vi "Kinetics camera control 1.vi"() -> ()   [LabVIEW 2020]
uses:
  C:/Users/Public/Documents/Photometrics/PMQI-LabViewSamples/Examples/2018/Dependencies/PVCamNET.dll
  PVCamNET.dll
panel:
  in  "stop":bool
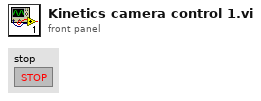
[diagram p1: front panel]
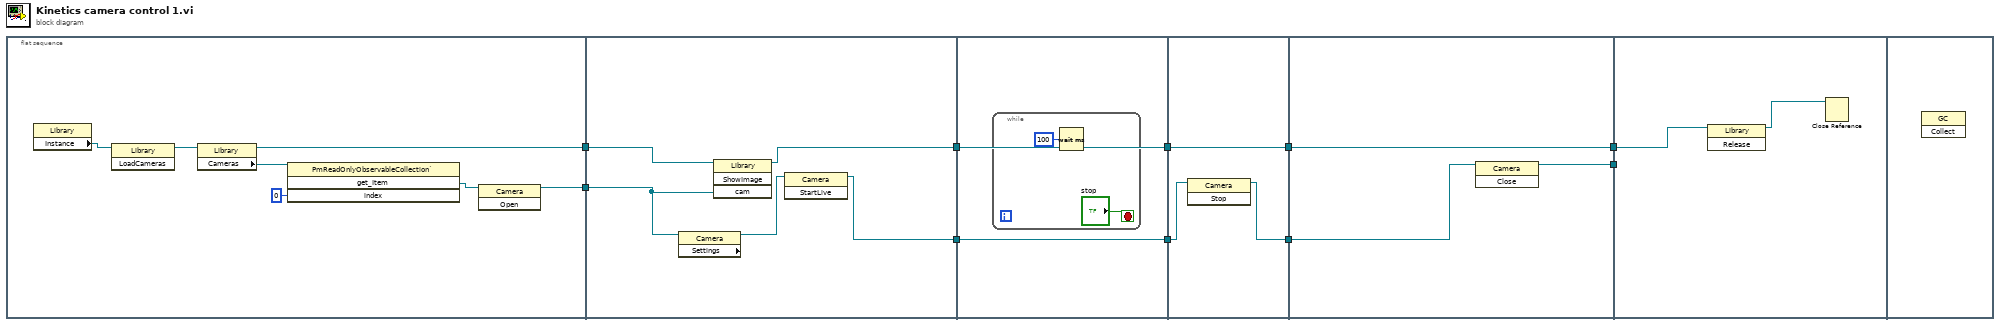
[diagram p0: block diagram]
diagram:
  n1 = flat-sequence {
    tunnel: [w14] -> w10
    tunnel: [w12] -> w9
    tunnel: w10 -> [w22]
    tunnel: [w19] -> w6
    tunnel: w9 -> [w21]
    tunnel: [w18] -> w5
    tunnel: w6 -> [w24]
    tunnel: [w24] -> w4
    tunnel: w5 -> [w23]
    tunnel: [w23] -> w2
    tunnel: w4 -> [w29]
    tunnel: [w29] -> w3
    tunnel: w2 -> [w28]
    tunnel: [w27] -> w1
    tunnel: w3 -> [w32]
    tunnel: [w32] -> w8
    tunnel: w1 -> [w31]
    tunnel: [w30] -> w7
    tunnel: w8 -> [w33]
    tunnel: w7 -> [_]
    frame #0 {
      n2 = property class="Library"() -> ("Instance"=w17:refnum<k24>)  [unwired: 2 in, 2 out]
      n3 = invoke class="Library" method="LoadCameras"(reference=w17) -> (reference out=w16:refnum<k24>)  [unwired: 2 in, 2 out]
      n4 = property class="Library"(reference=w16) -> (reference out=w14:refnum<k24>, "Cameras"=w15:refnum<k24>)  [unwired: 1 in, 1 out]
      n5 = invoke class="PmReadOnlyObservableCollection`" method="get_Item"(reference=w15, "index"=0) -> ("get_Item"=w13:refnum<k24>)  [unwired: 2 in, 3 out]
      n6 = invoke class="Camera" method="Open"(reference=w13) -> (reference out=w12:refnum<k24>)  [unwired: 2 in, 2 out]
    }
    frame #1 {
      n7 = property class="Camera" props=["Settings"](reference=w21) -> (reference out=w20:refnum<k24>)  [unwired: 1 in, 2 out]
      n8 = invoke class="Library" method="ShowImage"(reference=w22, "cam"=w21) -> (reference out=w19:refnum<k24>)  [unwired: 2 in, 3 out]
      n9 = invoke class="Camera" method="StartLive"(reference=w20) -> (reference out=w18:refnum<k24>)  [unwired: 2 in, 2 out]
    }
    frame #2 {
      n10 = while {
        stop <- "stop" stop-if-true
        n11 = Wait (ms)(milliseconds to wait=u32 100) -> ()  [unwired: 1 out]
      }
    }
    frame #3 {
      n12 = invoke class="Camera" method="Stop"(reference=w28) -> (reference out=w27:refnum<k24>)  [unwired: 2 in, 2 out]
    }
    frame #4 {
      n13 = invoke class="Camera" method="Close"(reference=w31) -> (reference out=w30:refnum<k24>)  [unwired: 2 in, 2 out]
    }
    frame #5 {
      n14 = invoke class="Library" method="Release"(reference=w33) -> (reference out=w34:refnum<k24>)  [unwired: 2 in, 2 out]
      n15 = Close Reference(reference=w34) -> ()  [unwired: 1 in, 1 out]
    }
    frame #6 {
      n16 = invoke class="GC" method="Collect"() -> ()  [unwired: 3 in, 3 out]
    }
  }
